vi "escapi_list_cameras.vi"(8 "error in (no error)":errorcluster) -> (0 "error out":errorcluster, 3 "Cam Names":string[](array[string]))   [LabVIEW 2022 SP3, in "Vision.lvlib"]
uses:
  Vision.lvlib
  Database/Database.lvlib
  bin/Vision.dll
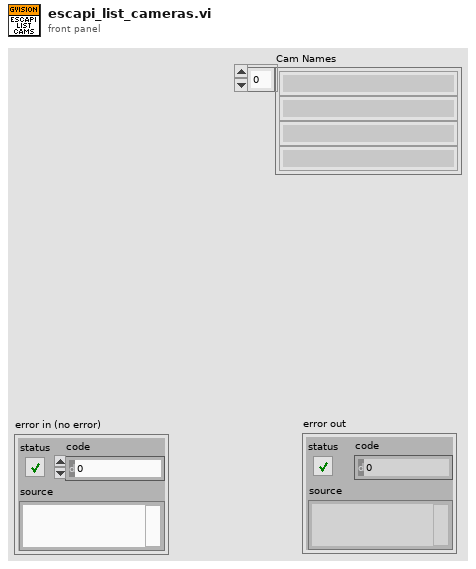
[diagram p1: front panel]
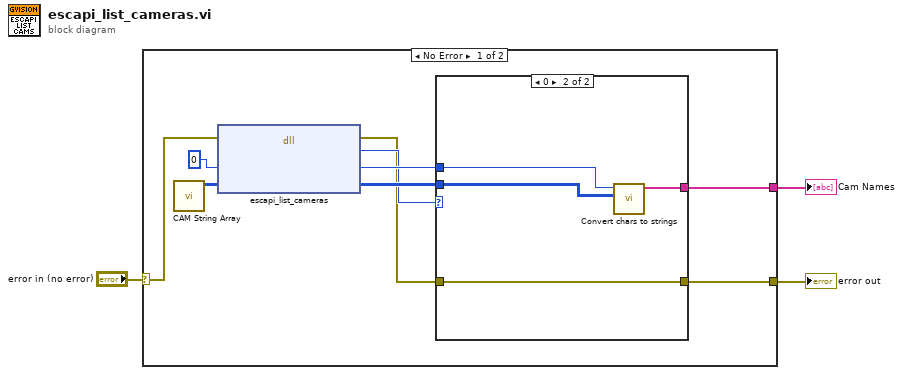
[diagram p0: block diagram]
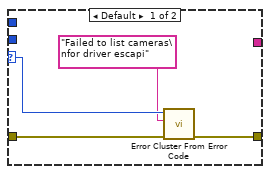
[diagram p2: hidden frame]
diagram:
  n1 = case shown="No Error" "error in (no error)" {
    selector: "error in (no error)" -> [w12 w21]
    tunnel: [w4 w21] -> w2
    tunnel: [w7 _] -> w1
    frame No Error {
      n2 = call "CAM String Array.vi"() -> ("CAM string array"=w10:i8[][])  [unwired: 11 in]
      n3 = dll-call lib="C:/Users/Caleb/Desktop/nebraska-silicon-lab/pixel-gantry-extra/LV/bin/Vision.dll" fn="escapi_list_cameras"(error in=w12, "n_cameras"=0, "names"=w10) -> (error out=w5:errorcluster, "return type"=w6:i32, "n_cameras"=w8:i32, "names"=w9:i8[][])  [unwired: 2 in, 1 out]
      n4 = case shown="0" w6 {
        selector: w6 -> [w14 _]
        tunnel: w9 -> [_ w20]
        tunnel: w8 -> [_ w19]
        tunnel: [_ w18] -> w7
        tunnel: w5 -> [w16 w17]
        tunnel: [w15 w17] -> w4
        frame Default {
          n5 = call <vilib>:"Error Cluster From Error Code.vi"("error in (no error)"=w16, "error message (\"\")"="Failed to list cameras\nfor driver escapi" ("error message (\"\")"), "error code (0)"=w14) -> ("error out"=w15:errorcluster)  [unwired: 6 in]
        }
        frame 0 {
          n6 = call "Convert chars to strings.vi"("Char Array"=w20, "Array Length"=w19) -> ("Strings"=w18:string[])  [unwired: 9 in]
        }
      }
    }
    frame Error {
    }
  }
  "error out" <- w2
  "Cam Names" <- w1
